vi "Send Progress and Message.vi"(8 "error in (no error)":errorcluster, 9 "Progress":i32, 10 "Message":string, 11 "ProgressBar in":refnum<class "ProgressBar.lvclass">) -> (0 "error out":errorcluster, 3 "ProgressBar out":refnum<class "ProgressBar.lvclass">)   [LabVIEW 2019, in "ProgressBar.lvclass"]
uses:
  ProgressBar.lvclass
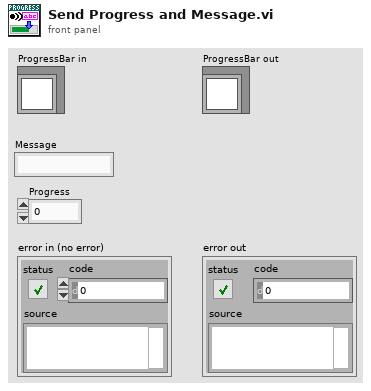
[diagram p1: front panel]
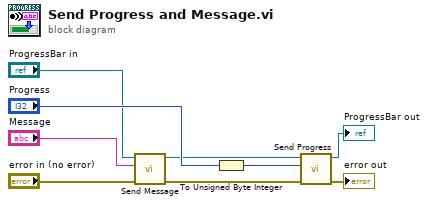
[diagram p0: block diagram]
diagram:
  n1 = call-dynamic "Send Message.vi"("error in (no error)"="error in (no error)", "Message"="Message", "ProgressBar"="ProgressBar in") -> ("error out"=w7:errorcluster, "ProgressBar out"=w2:refnum<class "ProgressBar.lvclass">)  [unwired: 7 in]
  n2 = To Unsigned Byte Integer(number="Progress") -> (unsigned 8bit integer=w1:u8)
  n3 = call "Send Progress.vi"("error in (no error)"=w7, "Send Progress"=w1, "ProgressBar"=w2) -> ("error out"=→"error out":errorcluster, "ProgressBar out"=→"ProgressBar out":refnum<class "ProgressBar.lvclass">)  [unwired: 7 in]
